vi "Set Mediator Settings.vi"(8 "error in (no error)":errorcluster, 10 "Mediator Settings":T1={"Remote"=FALSE, "IPAddress"="localhost", "Port"=8080}, 11 "Custom Device Ref in":T2 format="%.0x") -> (0 "error out":errorcluster, 3 "Custom Device Ref out":T2 format="%.0x")   [LabVIEW 2016, in "VeriStand Configuration Support.lvlib"]
uses:
  VeriStand Configuration Support.lvlib
  <vilib>/NI Veristand/Custom Device API/Custom Device Item Ref.ctl
  Mediator Settings.ctl
  Constants.vi
  <vilib>/NI Veristand/Custom Device API/Set Item Property (Variant).vi
  <vilib>/NI Veristand/Custom Device API/Custom Device API.lvlib
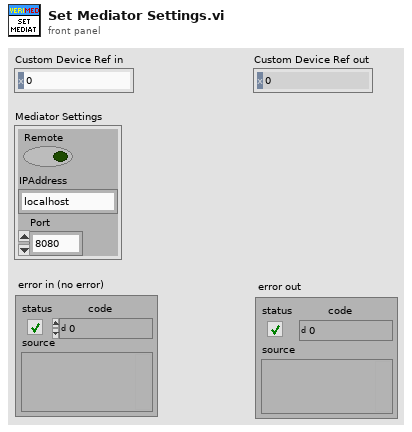
[diagram p1: front panel]
types:
  T1 = typedef "VeriStand Configuration Support.lvlib/Mediator Settings.ctl" = cluster{"Remote":bool, "IPAddress":string, "Port":u16}
  T2 = typedef "Custom Device API.lvlib/Custom Device Item Ref.ctl" = u64
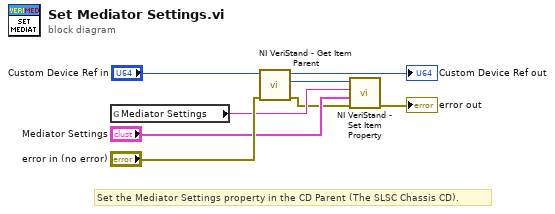
[diagram p0: block diagram]
diagram:
  # "Set the Mediator Settings property in the CD Parent (The SLSC Chassis CD)."
  n1 = global read "Constants.vi" "Mediator Settings"() -> (w3:string)
  n2 = call <vilib>:"NI VeriStand - Get Item Parent.vi"("error in (no error)"="error in (no error)", "Item Ref in"="Custom Device Ref in") -> ("error out"=w1:errorcluster, "Parent Ref"=w2:T2, "Item Ref out"=→"Custom Device Ref out":T2)  [unwired: 6 in, 1 out]
  n3 = call-poly <vilib>:"NI VeriStand - Set Item Property.vi"("error in (no error)"=w1, "Value"="Mediator Settings", "Property Name"=w3, "Item Ref in"=w2) -> ("error out"=→"error out":errorcluster)  [unwired: 5 in, 2 out]
